vi "Motor-Init.vi"() -> ()   [LabVIEW 2009]
panel:
  in  "Motor":string="PI1-M2-THETA"
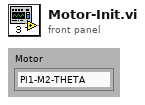
[diagram p1: front panel]
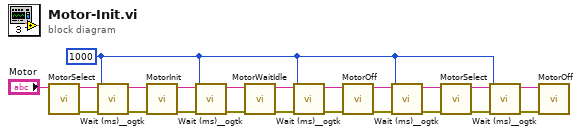
[diagram p0: block diagram]
diagram:
  w1 = u32 1000 ("milliseconds to wait")
  n1 = call "MotorSelect.vi"("Motor"="Motor") -> ("Motor out"=w16:string, "error out"=w11:errorcluster)  [unwired: 1 in, 6 out]
  n2 = call <userlib>:"Wait (ms)__ogtk.vi"("error in (no error)"=w11, "milliseconds to wait"=w1) -> ("error out"=w10:errorcluster)  [unwired: 1 in, 8 out]
  n3 = call "MotorInit.vi"("Motor"=w16, "error in (no error)"=w10) -> ("Motor out"=w13:string, "error out"=w9:errorcluster)  [unwired: 6 out]
  n4 = call <userlib>:"Wait (ms)__ogtk.vi"("error in (no error)"=w9, "milliseconds to wait"=w1) -> ("error out"=w8:errorcluster)  [unwired: 1 in, 8 out]
  n5 = call "MotorWaitIdle.vi"("Motor"=w13, "error in (no error)"=w8) -> ("Motor out"=w12:string, "error out"=w7:errorcluster)  [unwired: 6 out]
  n6 = call <userlib>:"Wait (ms)__ogtk.vi"("error in (no error)"=w7, "milliseconds to wait"=w1) -> ("error out"=w6:errorcluster)  [unwired: 1 in, 8 out]
  n7 = call "MotorOff.vi"("Motor"=w12, "error in (no error)"=w6) -> ("Motor out"=w15:string, "error out"=w5:errorcluster)  [unwired: 6 out]
  n8 = call <userlib>:"Wait (ms)__ogtk.vi"("error in (no error)"=w5, "milliseconds to wait"=w1) -> ("error out"=w4:errorcluster)  [unwired: 1 in, 8 out]
  n9 = call "MotorSelect.vi"("Motor"=w15, "error in (no error)"=w4) -> ("Motor out"=w14:string, "error out"=w3:errorcluster)  [unwired: 6 out]
  n10 = call <userlib>:"Wait (ms)__ogtk.vi"("error in (no error)"=w3, "milliseconds to wait"=w1) -> ("error out"=w2:errorcluster)  [unwired: 1 in, 8 out]
  n11 = call "MotorOff.vi"("Motor"=w14, "error in (no error)"=w2) -> ()  [unwired: 8 out]
